vi "SetMapPosition.vi"(0 "object in":refnum<class "Battleship.lvclass">, 2 "MapPosition":T1, 5 "error in (no error)":errorcluster) -> (14 "object out":refnum<class "Battleship.lvclass">, 19 "error out":errorcluster)   [LabVIEW 2015, in "Battleship.lvclass"]
doc: "Translates the ship footprint into map coordinates relative to the MapPosition input."
uses:
  Battleship.lvclass
  TypDefs/Coordinates.ctl
  Battleship.lvclass/Battleship.ctl
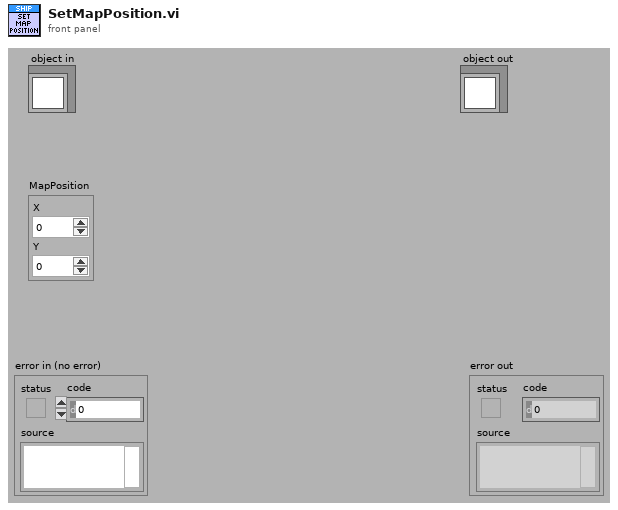
[diagram p1: front panel]
types:
  T1 = typedef "Coordinates.ctl" = cluster{"X":i32, "Y":i32}
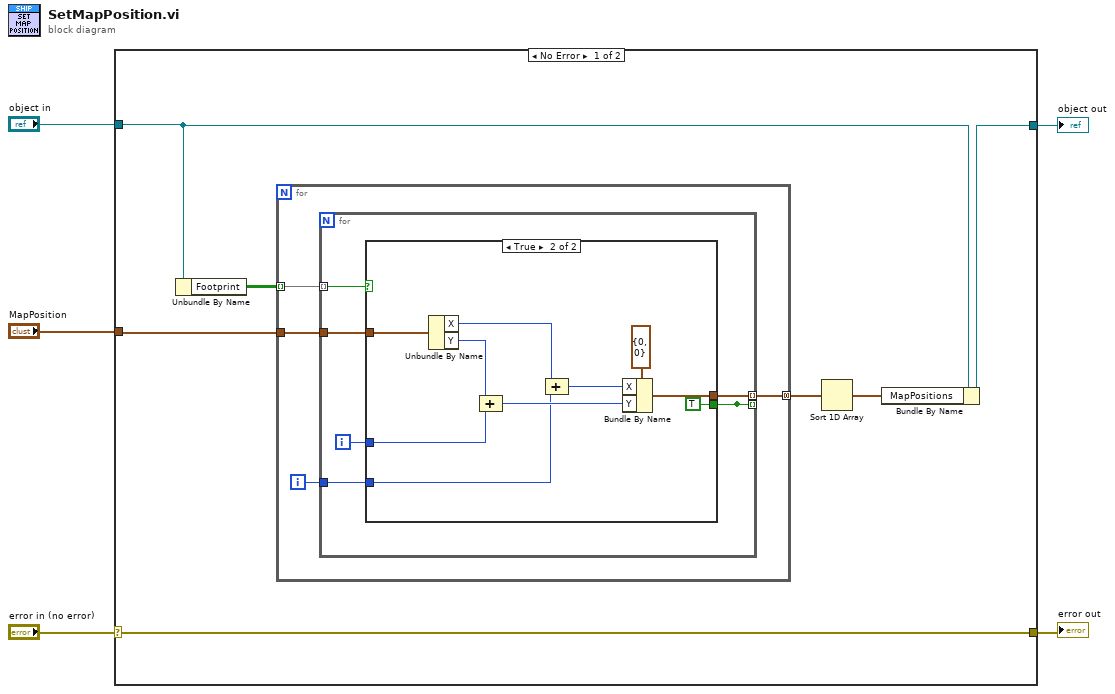
[diagram p0: block diagram]
diagram:
  n1 = case shown="No Error" "error in (no error)" {
    selector: "error in (no error)" -> [w12 w35]
    tunnel: [w12 w35] -> w4
    tunnel: [w11 w34] -> w2
    tunnel: "object in" -> [w10 w34]
    tunnel: "MapPosition" -> [w8 _]
    frame No Error {
      n2 = Unbundle By Name(w10) -> ("Footprint"=w9:bool[][])
      n3 = for {
        tunnel: w9 -> [w16] mode=indexing
        tunnel: w8 -> [w15]
        tunnel: [w13] -> w7 mode=concatenating
        i -> [w14]
        n4 = for {
          tunnel: w16 -> [w22] mode=indexing
          tunnel: w15 -> [w21]
          tunnel: w14 -> [w19]
          tunnel: [w18] -> w13 mode=indexing if=w17
          tunnel: [w17] -> _ mode=indexing
          i -> [w20]
          n5 = case shown="True" w22 {
            selector: w22 -> [w23 _]
            tunnel: w21 -> [_ w33]
            tunnel: w20 -> [_ w25]
            tunnel: w19 -> [_ w26]
            tunnel: [_ w28] -> w18
            tunnel: [w23 TRUE] -> w17
            frame False {
            }
            frame True {
              n6 = Unbundle By Name(w33) -> ("X"=w32:i32, "Y"=w31:i32)
              n7 = Compound Arithmetic op=ADD(w31, w25) -> (w29:i32)
              n8 = Compound Arithmetic op=ADD(w32, w26) -> (w30:i32)
              n9 = Bundle By Name(cluster=T1 {"X"=0, "Y"=0} ("Coordinates"), "X"=w30, "Y"=w29) -> (w28:T1)
            }
          }
        }
      }
      n10 = Sort 1D Array(array=w7) -> (sorted array=w6:T1[])
      n11 = Bundle By Name(cluster=w10, "MapPositions"=w6) -> (w11:refnum<class "Battleship.lvclass">)
    }
    frame Error {
    }
  }
  "error out" <- w4
  "object out" <- w2
